vi "Set 2D Array Double.vi"(5 "use temporary file? (F)":bool, 8 "error in":errorcluster, 9 "value":dbl[][](array[numeric]), 10 "variable name":string, 11 "GOLPI ref. in":T1={"pipe handle"={"lv_proc.dll file path"=path "", "process instance handle"=[], "debug mode"=FALSE, "debug data"=[]}, "fast read timeout [ms]"=500, "fast read settle time [ms]"=10, "fast read to multiple [ms]"=1, "max elements per input line"=100, "slow read timeout [ms]"=5000, "stdin double format specifier"="%_16e", "max elements per stdout output column"=100, "console mode bitstream"=FALSE, "bitstream first read timeout [ms]"=1000, "bitstream read timeout [ms]"=50, "struct transfer possible"=FALSE, "matlab mode"=FALSE, "var pipe write timeout [ms]"=5000, "variable pipe mode"=FALSE, "variable pipe buffer size [Bytes]"=10000000, "variable pipe block size [Bytes]"=1000000} {"variable pipe block size [Bytes]" format="%.0p"; "variable pipe buffer size [Bytes]" format="%.0p"}) -> (0 "error out":errorcluster, 3 "GOLPI ref. out":T1={"pipe handle"={"lv_proc.dll file path"=path "", "process instance handle"=[], "debug mode"=FALSE, "debug data"=[]}, "fast read timeout [ms]"=500, "fast read settle time [ms]"=10, "fast read to multiple [ms]"=1, "max elements per input line"=100, "slow read timeout [ms]"=5000, "stdin double format specifier"="%_16e", "max elements per stdout output column"=100, "console mode bitstream"=FALSE, "bitstream first read timeout [ms]"=1000, "bitstream read timeout [ms]"=50, "struct transfer possible"=FALSE, "matlab mode"=FALSE, "var pipe write timeout [ms]"=5000, "variable pipe mode"=FALSE, "variable pipe buffer size [Bytes]"=10000000, "variable pipe block size [Bytes]"=1000000} {"variable pipe block size [Bytes]" format="%.0p"; "variable pipe buffer size [Bytes]" format="%.0p"})   [LabVIEW 2020, in "GOLPI library.lvlib"]
doc: "Part of polymorph Set Variable.vi"
uses:
  GOLPI library.lvlib
  Public/GOLPI reference Type Def.ctl
  LV Process source distribution/Pipe Handle.ctl
  LV Process source distribution/LV Process library.lvlib
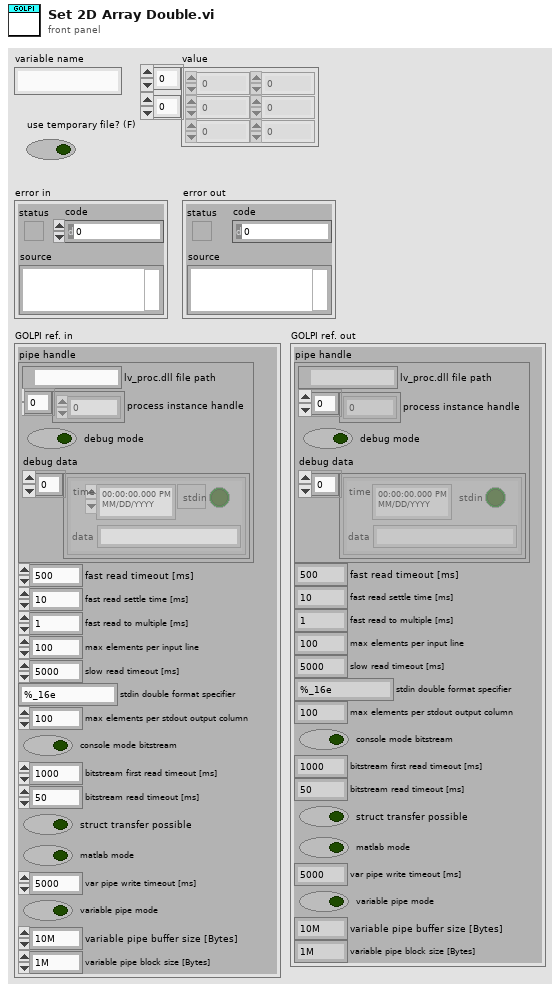
[diagram p1: front panel]
types:
  T1 = typedef "GOLPI library.lvlib/GOLPI reference Type Def.ctl" = cluster{"pipe handle":T2, "fast read timeout [ms]":u32, "fast read settle time [ms]":u32, "fast read to multiple [ms]":u32, "max elements per input line":u32, "slow read timeout [ms]":u32, "stdin double format specifier":string, "max elements per stdout output column":u32, "console mode bitstream":bool, "bitstream first read timeout [ms]":u32, "bitstream read timeout [ms]":u32, "struct transfer possible":bool, "matlab mode":bool, "var pipe write timeout [ms]":u32, "variable pipe mode":bool, "variable pipe buffer size [Bytes]":u32, "variable pipe block size [Bytes]":u32}
  T2 = typedef "LV Process library.lvlib/Pipe Handle.ctl" = cluster{"lv_proc.dll file path":path, "process instance handle":u32[], "debug mode":bool, "debug data":cluster{"time":timestamp, "stdin":bool, "data":string}[]}
  T3 = typedef "GOLPI library.lvlib/Transfer Mode.ctl" = enum16{"Matlab", "stdio", "temp file", "bitstream", "pipe"}
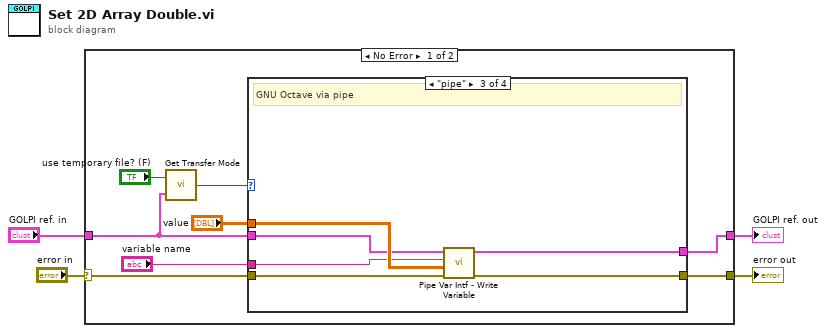
[diagram p0: block diagram]
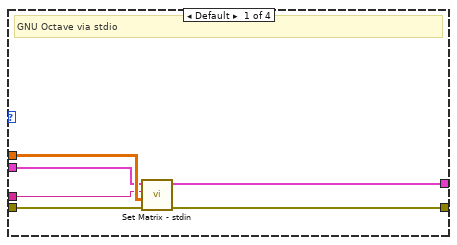
[diagram p2: hidden frame]
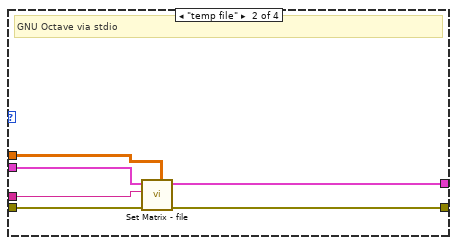
[diagram p3: hidden frame]
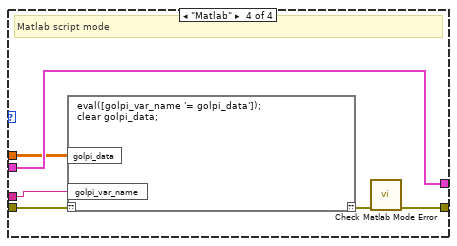
[diagram p4: hidden frame]
diagram:
  n1 = case shown="No Error" "error in" {
    selector: "error in" -> [w10 w38]
    tunnel: [w9 w38] -> w4
    tunnel: "GOLPI ref. in" -> [w6 w37]
    tunnel: [w8 w37] -> w1
    frame No Error {
      n2 = call "Get Transfer Mode.vi"("GOLPI ref."=w6, "use temporary file? (F)"="use temporary file? (F)") -> ("mode"=w5:T3)
      n3 = case shown="\"pipe\"" w5 {
        tunnel: "value" -> [w18 w24 w30 w34]
        tunnel: "variable name" -> [w17 w23 w29 w33]
        tunnel: w10 -> [w16 w22 w28 w36]
        tunnel: [w15 w21 w27 w31] -> w9
        tunnel: w6 -> [w14 w20 w26 w35]
        tunnel: [w13 w19 w25 w35] -> w8
        frame Default {
          # "GNU Octave via stdio"
          n4 = call "Set Matrix - stdin.vi"("error in"=w16, "value"=w18, "variable name"=w17, "GOLPI ref. in"=w14) -> ("error out"=w15:errorcluster, "GOLPI ref. out"=w13:T1)  [unwired: 6 in]
        }
        frame "temp file" {
          # "GNU Octave via stdio"
          n5 = call "Set Matrix - file.vi"("double array"=w24, "error in (no error)"=w22, "variable name"=w23, "GOLPI ref. in"=w20) -> ("error out"=w21:errorcluster, "GOLPI ref. out"=w19:T1)  [unwired: 6 in]
        }
        frame "pipe" {
          # "GNU Octave via pipe"
          n6 = call "Pipe Var Intf - Write Variable.vi"("error in (no error)"=w28, "data in"=w30, "variable name"=w29, "GOLPI ref. in"=w26) -> ("error out"=w27:errorcluster, "GOLPI ref. out"=w25:T1)  [unwired: 6 in]
        }
        frame "Matlab" {
          # "Matlab script mode"
          n7 = script code="eval([golpi_var_name '= golpi_data']);\nclear golpi_data;"("??"=w36, "golpi_var_name"=w33, "golpi_data"=w34) -> ("??"=w32:errorcluster)
          n8 = call "Check Matlab Mode Error.vi"("error in"=w32) -> ("error out"=w31:errorcluster)  [unwired: 10 in]
        }
      }
    }
    frame Error {
    }
  }
  "error out" <- w4
  "GOLPI ref. out" <- w1
